vi "MOPX1 Engine.vi"(6 "Due Dates":u16[](array[numeric]), 7 "Job Selection Rule":T1, 8 "Main Parent Job Completion Times":u16[](array[numeric]), 9 "Main Parent  MO4J":u16[][](array[numeric]), 10 "Secondary Parent Schedule":u16[](array[numeric]), 11 "Main Parent Schedule":u16[](array[numeric])) -> (3 "Child Schedule":u16[](array[numeric]))   [LabVIEW 2013, in "GA.lvclass"]
uses:
  GA.lvclass
  Controls/MPOX1 Operation Selection Rule.ctl
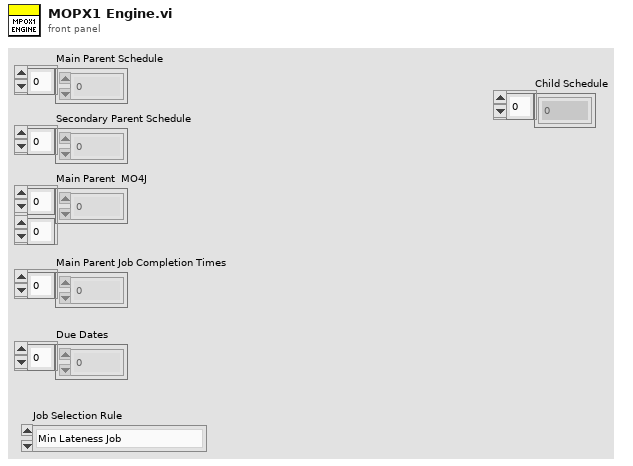
[diagram p1: front panel]
types:
  T1 = typedef "GA.lvclass/MPOX1 Operation Selection Rule.ctl" = enum16{"Min Lateness Job", "Random Job"}
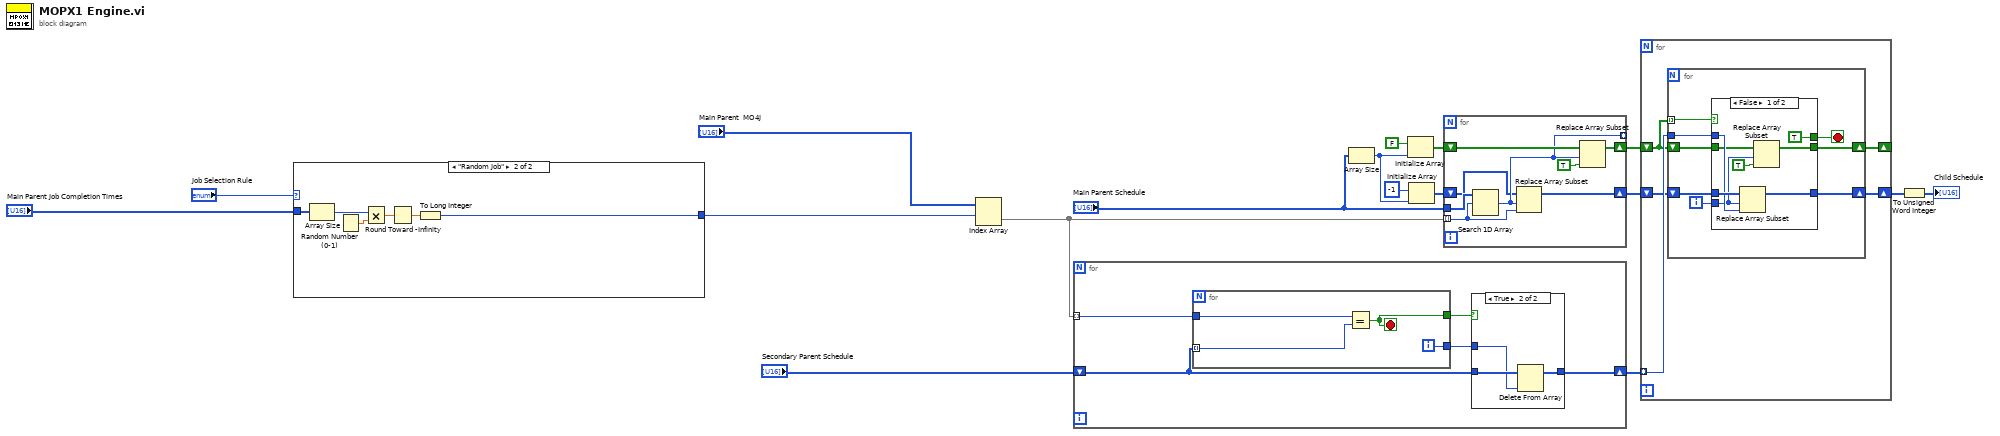
[diagram p0: block diagram]
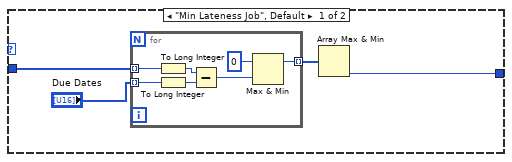
[diagram p2: hidden frame]
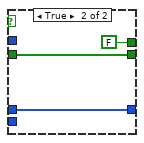
[diagram p3: hidden frame]
diagram:
  n1 = case shown="\"Random Job\"" "Job Selection Rule" {
    tunnel: "Main Parent Job Completion Times" -> [w20 w34]
    tunnel: [w18 w29] -> w13
    frame "Min Lateness Job", Default {
      n2 = for {
        tunnel: w20 -> [w25] mode=indexing
        tunnel: "Due Dates" -> [w24] mode=indexing
        tunnel: [w26] -> w19 mode=indexing
        n3 = To Long Integer(number=w25) -> (32bit integer=w22:i32)
        n4 = To Long Integer(number=w24) -> (32bit integer=w23:i32)
        n5 = Subtract(x=w22, y=w23) -> (x-y=w28:i32)
        n6 = Max & Min(x=0, y=w28) -> (max(x,y)=w26:i32)  [unwired: 1 out]
      }
      n7 = Array Max & Min(array=w19) -> (min index (indices)=w18:i32)  [unwired: 3 out]
    }
    frame "Random Job" {
      n8 = Array Size(array=w34) -> (size(s)=w33:i32)
      n9 = Random Number (0-1)() -> (number: 0 to 1=w32:dbl)
      n10 = Multiply(x=w33, y=w32) -> (x*y=w31:dbl)
      n11 = Round Toward -Infinity(1:w31) -> (0:w30:dbl)
      n12 = To Long Integer(number=w30) -> (32bit integer=w29:i32)
    }
  }
  n13 = Index Array(array="Main Parent  MO4J", index (row)=w13) -> (element=w12:u16[])  [unwired: 1 in]
  n14 = for {
    tunnel: w12 -> [w39] mode=indexing
    shift-right: [w36] -> w3
    shift-left: "Secondary Parent Schedule" -> [w38]
    n15 = for {
      tunnel: w38 -> [w46] mode=indexing
      tunnel: w39 -> [w47]
      tunnel: [w45] -> w37
      tunnel: [w44] -> w35
      i -> [w45]
      stop <- w44 stop-if-true
      n16 = Equal?(x=w47, y=w46) -> (x = y?=w44:bool)
    }
    n17 = case shown="True" w35 {
      tunnel: w38 -> [w40 w43]
      tunnel: w37 -> [_ w42]
      tunnel: [w40 w41] -> w36
      frame False {
      }
      frame True {
        n18 = Delete From Array(array=w43, index=w42) -> (array with subset deleted=w41:u16[])  [unwired: 1 in, 1 out]
      }
    }
  }
  n19 = Array Size(array="Main Parent Schedule") -> (size(s)=w9:i32)
  n20 = Initialize Array(FALSE, w9) -> (w11:bool[])
  n21 = Initialize Array(-1, w9) -> (w7:i32[])
  n22 = for {
    tunnel: "Main Parent Schedule" -> [w55]
    tunnel: w12 -> [w51] mode=indexing
    tunnel: [w52] -> _ mode=indexing
    shift-right: [w48] -> w5
    shift-left: w11 -> [w54]
    shift-right: [w49] -> w4
    shift-left: w7 -> [w50]
    n23 = Search 1D Array(1D array=w55, element=w51) -> (index of element=w52:i32)  [unwired: 1 in]
    n24 = Replace Array Subset(array=w50, new element=w51, index=w52) -> (w49:i32[])
    n25 = Replace Array Subset(array=w54, new element=TRUE ("new element/subarray"), index=w52) -> (w48:bool[])
  }
  n26 = for {
    tunnel: w3 -> [w60] mode=indexing
    shift-right: [w58] -> w2
    shift-left: w4 -> [w59]
    shift-right: [w56] -> _
    shift-left: w5 -> [w57]
    n27 = for {
      tunnel: w57 -> [w68] mode=indexing
      tunnel: w60 -> [w65]
      shift-right: [w66] -> w58
      shift-left: w59 -> [w67]
      shift-right: [w62] -> w56
      shift-left: w57 -> [w63]
      i -> [w64]
      stop <- w61 stop-if-true
      n28 = case shown="False" w68 {
        tunnel: w67 -> [w76 w79]
        tunnel: [w74 w79] -> w66
        tunnel: w65 -> [w75 _]
        tunnel: w64 -> [w72 _]
        tunnel: w63 -> [w73 w78]
        tunnel: [w70 w78] -> w62
        tunnel: [TRUE FALSE] -> w61
        frame False {
          n29 = Replace Array Subset(array=w76, new element=w75, index=w72) -> (w74:i32[])
          n30 = Replace Array Subset(array=w73, new element=TRUE ("new element/subarray"), index=w72) -> (w70:bool[])
        }
        frame True {
        }
      }
    }
  }
  n31 = To Unsigned Word Integer(number=w2) -> (unsigned 16bit integer=→"Child Schedule":u16[])
